vi "populate_settings_combo.vi"(5 "trigger value change event?":bool=TRUE, 6 "force default settings":bool, 7 "force settings":string, 8 "error in (no error)":errorcluster, 10 "combo box ref":refnum<vi>, 11 "GenericPlugin in":refnum<class "GenericComponent.lvclass">) -> (0 "error out":errorcluster, 3 "GenericPlugin out":refnum<class "GenericComponent.lvclass">)   [LabVIEW 2010, in "GenericComponent.lvclass"]
uses:
  GenericComponent.lvclass
  <vilib>/regexp/Match Regular Expression.xnode
panel:
  # "Value set after populating the settings combo box:\n\n1. Settings specified by \"force settings\" input.\n2. Default settings present in settings folder, if \"force default settings\"=true or internal settings not specified.\n3. Internal settings, if specifed\n4. user-defined otherwise"
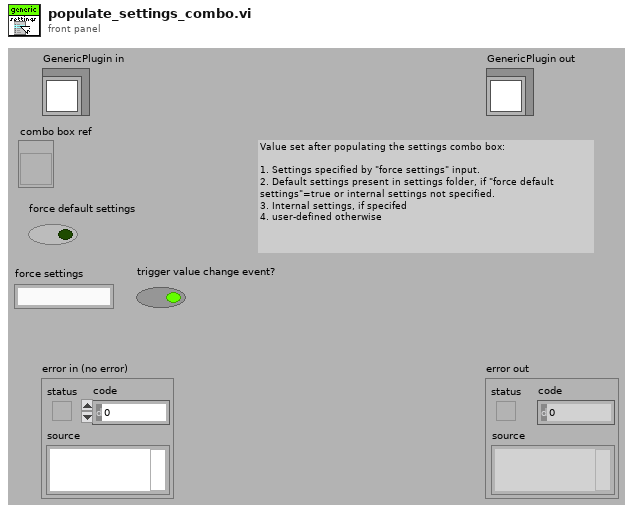
[diagram p1: front panel]
types:
  T1 = typedef "plugin_specification.ctl" = cluster{"class path":string, "configuration":string, "label":string, "settings name":string}
  T2 = cluster{"before match":string, "before match":string}
  T3 = cluster{"before match":string, "before match":string}[]
  T4 = cluster{"force settings":string, "force settings":string}
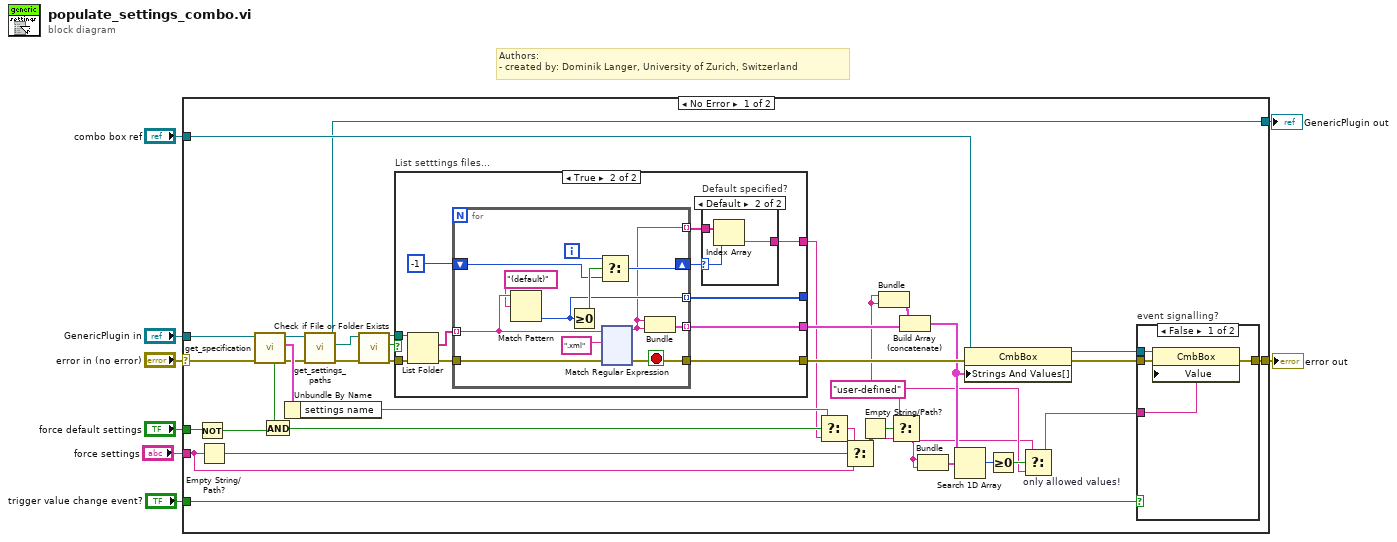
[diagram p0: block diagram]
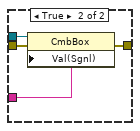
[diagram p2: hidden frame]
diagram:
  # "Authors: \n- created by: Dominik Langer, University of Zurich, Switzerland"
  n1 = case shown="No Error" "error in (no error)" {
    selector: "error in (no error)" -> [w25 w193]
    tunnel: [w44 w193] -> w8
    tunnel: "combo box ref" -> [w43 _]
    tunnel: "GenericPlugin in" -> [w24 w192]
    tunnel: [w33 w192] -> w5
    tunnel: "force default settings" -> [w39 _]
    tunnel: "force settings" -> [w20 _]
    tunnel: "trigger value change event?" -> [w9 _]
    frame No Error {
      w13 = "user-defined"
      n2 = Not(x=w39) -> (.not. x?=w38:bool)
      n3 = Empty String/Path?(string/path=w20) -> (empty?=w21:bool)
      n4 = call-dynamic "get_specification.vi"("error in (no error)"=w25, "GenericPlugin in"=w24) -> ("error out"=w35:errorcluster, "component specification"=w41:T1, "GenericPlugin out"=w34:refnum<class "GenericComponent.lvclass">, "settings specified?"=w37:bool)  [unwired: 6 in]
      n5 = And(x=w37, y=w38) -> (x .and. y?=w36:bool)
      n6 = Unbundle By Name(w41) -> ("settings name"=w40:string)
      n7 = call-dynamic "get_settings_paths.vi"("error in (no error)"=w35, "GenericComponent in"=w34) -> ("error out"=w30:errorcluster, "settings folder for a specific component"=w22:path, "GenericComponent out"=w33:refnum<class "GenericComponent.lvclass">)  [unwired: 4 in, 3 out]
      n8 = call <vilib>:"Check if File or Folder Exists.vi"("error in (no error)"=w30, "path"=w22) -> ("error out"=w29:errorcluster, "file or folder exists?"=w28:bool, "dup path"=w31:path)  [unwired: 7 in]
      n9 = case "List setttings files..." shown="True" w28 {
        tunnel: [w54 w62] -> w32
        tunnel: w31 -> [_ w65]
        tunnel: w29 -> [w54 w64]
        tunnel: [_ w61] -> w27
        tunnel: [_ w58] -> w23
        tunnel: [_ w56] -> _
        frame False {
        }
        frame True {
          n10 = List Folder(path=w65, error in=w64) -> (filenames=w59:string[], error out=w63:errorcluster)  [unwired: 2 in, 2 out]
          n11 = for {
            tunnel: w59 -> [w77] mode=indexing
            tunnel: w63 -> [w80]
            tunnel: [w79] -> w62
            tunnel: [w69] -> w61 mode=indexing
            shift-right: [w75] -> w57
            shift-left: -1 -> [w73]
            tunnel: [w72] -> w56 mode=indexing
            tunnel: [w70] -> w55 mode=indexing
            i -> [w71]
            stop <- w79 stop-if-true
            n12 = Match Pattern(string=w77, regular expression="(default)") -> (offset past match=w72:i32)  [unwired: 1 in, 3 out]
            n13 = Greater Or Equal To 0?(x=w72) -> (x >= 0?=w74:bool)
            n14 = Select(t=w71, s=w74, f=w73) -> (s? t:f=w75:i32)
            n15 = xnode "Match Regular Expression"("input string"=w77, "regular expression"=".xml", "error in"=w80) -> ("before match"=w70:string, "error out"=w79:errorcluster)  [unwired: 3 in, 3 out]
            n16 = Bundle("before match"=w70, "before match"=w70) -> (w69:T2)  [unwired: 1 in]
          }
          n17 = case "Default specified?" shown="Default" w57 {
            selector: w57 -> [_ w66]
            tunnel: w55 -> [_ w68]
            tunnel: [_ w67] -> w58
            frame -1 {
              # "No..."
            }
            frame Default {
              n18 = Index Array(array=w68, index=w66) -> (element=w67:string)
            }
          }
        }
      }
      n19 = Select(t=w40, s=w36, f=w23) -> (s? t:f=w19:string)
      n20 = Select(t=w19, s=w21, f=w20) -> (s? t:f=w18:string)
      n21 = Empty String/Path?(string/path=w18) -> (empty?=w26:bool)
      n22 = Bundle(w13, w13) -> (w12:cluster{string, string})  [unwired: 1 in]
      n23 = Select(t=w13, s=w26, f=w18) -> (s? t:f=w10:string)
      n24 = Build Array (concatenate)(w12, w27) -> (w17:T3)
      n25 = Bundle("force settings"=w10, "force settings"=w10) -> (w11:T4)  [unwired: 1 in]
      n26 = Search 1D Array(1D array=w17, element=w11) -> (index of element=w16:i32)  [unwired: 1 in]
      n27 = property class="CmbBox"(reference=w43, error in=w32, "Strings And Values[]"=w17) -> (reference out=w42:refnum<vi>, error out=w45:errorcluster)
      n28 = Greater Or Equal To 0?(x=w16) -> (x >= 0?=w15:bool)
      n29 = Select "only allowed values!"(t=w10, s=w15, f=w13) -> (s? t:f=w14:string)
      n30 = case "event signalling?" shown="False" w9 {
        tunnel: w45 -> [w47 w53]
        tunnel: [w46 w52] -> w44
        tunnel: w42 -> [w48 w51]
        tunnel: w14 -> [w49 w50]
        frame False {
          n31 = property class="CmbBox"(reference=w48, error in=w47, "Value"=w49) -> (error out=w46:errorcluster)  [unwired: 1 out]
        }
        frame True {
          n32 = property class="CmbBox"(reference=w51, error in=w53, "Val(Sgnl)"=w50) -> (error out=w52:errorcluster)  [unwired: 1 out]
        }
      }
    }
    frame Error {
    }
  }
  "error out" <- w8
  "GenericPlugin out" <- w5
